vi "Keithley 2000 Series.vi"(2 "Point #":i32, 3 "Instrument Address":refnum<visa-resource-name>) -> (0 "Stop":bool, 1 "Measurement":dbl[](array[numeric]) format="%.6e")   [LabVIEW 2021]
doc: "This VI reads a single reading from a Keithley 2001 multimeter. The stop boolean is always false. If no reading is obtained a single zero is returned.\nScott Hannahs, NHMFL-FSU, Nov 1993"
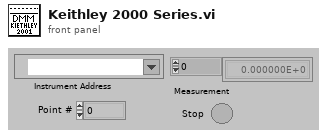
[diagram p1: front panel]
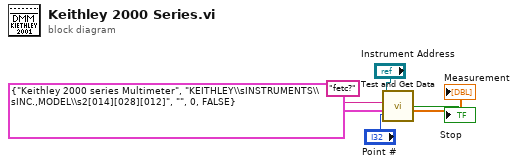
[diagram p0: block diagram]
diagram:
  n1 = call "Test and Get Data.vi"("Point #"="Point #", "Instrument Info"=cluster{string, string, string, u32, bool} {"Keithley 2000 series Multimeter", "KEITHLEY\\sINSTRUMENTS\\sINC.,MODEL\\s2[014][028][012]", "", 0, FALSE}, "Command String"="fetc?", "VISA Sesson"="Instrument Address") -> ("Measurement"=→"Measurement":dbl[], "Stop"=→"Stop":bool)  [unwired: 2 in, 3 out]
